vi "restrictoutput.vi"(11 "Input":dbl) -> (1 "Hig":bool, 2 "Output":u16, 3 "Low":bool)   [LabVIEW 2018, in "pid-toolkit.lvlib"]
uses:
  pid-toolkit.lvlib
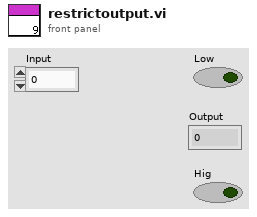
[diagram p1: front panel]
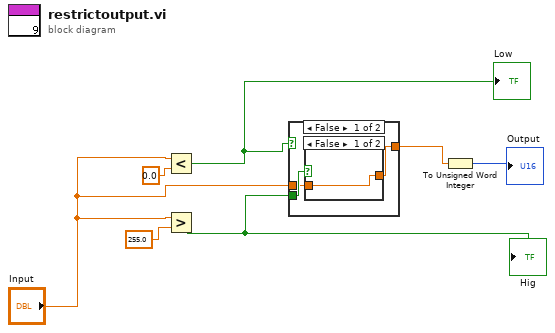
[diagram p0: block diagram]
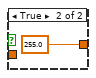
[diagram p2: hidden frame]
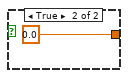
[diagram p3: hidden frame]
diagram:
  n1 = Less?(x="Input", y=0.0) -> (x < y?=w3:bool)
  "Low" <- w3
  n2 = Greater?(x="Input", y=255.0) -> (0:w4:bool)
  "Hig" <- w4
  n3 = case shown="False" w3 {
    tunnel: w4 -> [w10 _]
    tunnel: [w9 0.0 ("y")] -> w6
    tunnel: "Input" -> [w8 _]
    frame False {
      n4 = case shown="False" w10 {
        tunnel: [w11 255.0 ("y")] -> w9
        tunnel: w8 -> [w11 _]
        frame False {
        }
        frame True {
        }
      }
    }
    frame True {
    }
  }
  n5 = To Unsigned Word Integer(number=w6) -> (unsigned 16bit integer=→"Output":u16)
